vi "Do.vi"(8 "error in (no error)":errorcluster, 11 "AppLogger.Message.StartUp in":refnum<class "AppLogger.Message.StartUp.lvclass">) -> (0 "error out":errorcluster, 3 "AppLogger.Message.StartUp out":refnum<class "AppLogger.Message.StartUp.lvclass">)   [LabVIEW 2014, in "AppLogger.Message.StartUp.lvclass"]
uses:
  AppLogger.Message.StartUp.lvclass
  Message/Message.lvclass
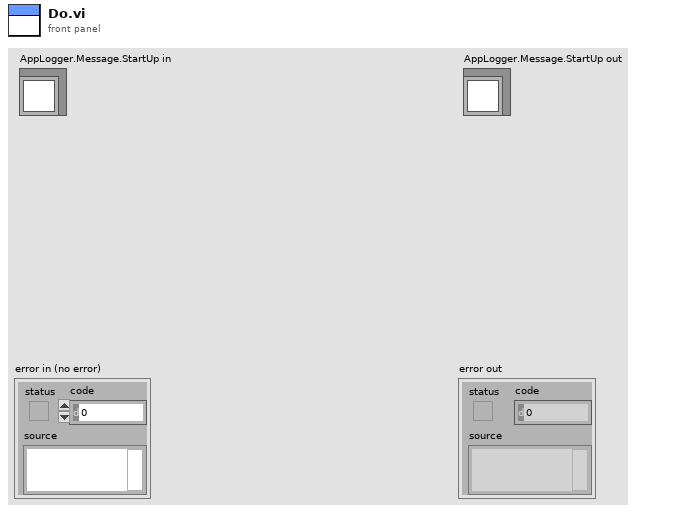
[diagram p1: front panel]
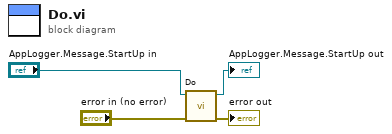
[diagram p0: block diagram]
diagram:
  n1 = call-parent "Do.vi"("error in (no error)"="error in (no error)", "Message in"="AppLogger.Message.StartUp in") -> ("error out"=→"error out":errorcluster, "Message out"=→"AppLogger.Message.StartUp out":refnum<class "AppLogger.Message.StartUp.lvclass">)  [unwired: 8 in]
